vi "Configure Output Range.vi"(0 "VISA resource name":refnum<visa-resource-name>, 5 "Function(0:Voltage)":u16(ring) items=["Voltage", "Current"], 7 "Output Range(0:Min)":u16(ring) items=["Min", "Max"], 11 "error in (no error)":errorcluster) -> (4 "VISA resource name out":refnum<visa-resource-name>, 15 "error out":errorcluster)   [LabVIEW 2021, in "Keithley 2200 Series.lvlib"]
doc: "Configure the Minimum and Maximum range for selected function.\n\nNote: Call the Enable Output.vi before Configure Output Range.vi"
uses:
  <instrlib>/Keithley 2200 Series/Keithley 2200 Series.lvlib
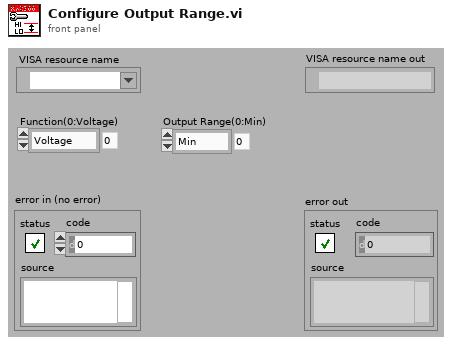
[diagram p1: front panel]
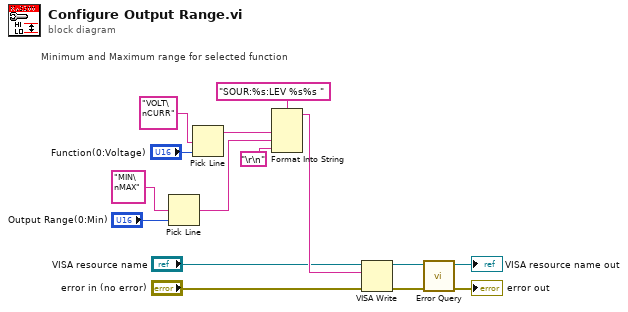
[diagram p0: block diagram]
diagram:
  # "Minimum and Maximum range for selected function"
  n1 = Pick Line(multi-line string="MIN\nMAX", line index="Output Range(0:Min)") -> (output string=w9:string)  [unwired: 1 out]
  n2 = Pick Line(multi-line string="VOLT\nCURR" ("format string"), line index="Function(0:Voltage)") -> (output string=w6:string)  [unwired: 1 out]
  n3 = Format Into String(format string="SOUR:%s:LEV %s%s ", w6, w9, "\r\n") -> (resulting string=w5:string)  [unwired: 2 in, 1 out]
  n4 = VISA Write(VISA resource name="VISA resource name", write buffer=w5, error in (no error)="error in (no error)") -> (VISA resource name out=w15:refnum<visa-resource-name>, error out=w14:errorcluster)  [unwired: 1 out]
  n5 = call <instrlib>:"Error Query.vi"("error in (no error)"=w14, "VISA resource name"=w15) -> ("error out"=→"error out":errorcluster, "VISA resource name out"=→"VISA resource name out":refnum<visa-resource-name>)  [unwired: 8 out]
